vi "AMC e.bloxx Write.vi"(8 "error in (no error)":errorcluster, 9 "Module Command":string, 10 "Module Address":i32, 11 "VISA Resource Name":refnum<visa-resource-name>) -> (0 "error out":errorcluster, 3 "VISA Resource Name out":refnum<visa-resource-name>)   [LabVIEW 2016]
doc: "<B>AMC - Analytik & Messtechnik GmbH Chemnitz</B>\n\nLabVIEW Drivers for e.bloxx series from Gantner Instruments\n\nThis VI is a driver subroutine and should not be used in an application. It assembles a module command string out of the parameters and writes it to the serial interface specified in <B>VISA Resource Name</B>."
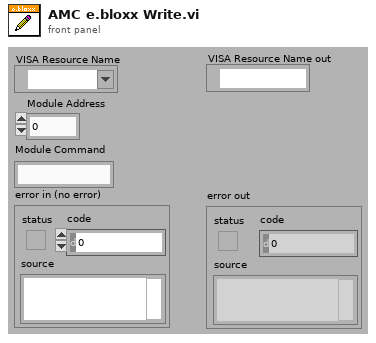
[diagram p1: front panel]
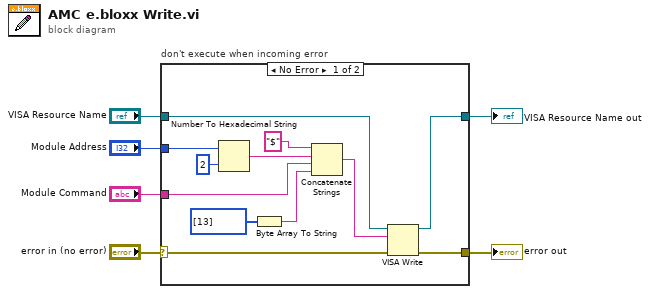
[diagram p0: block diagram]
diagram:
  n1 = case "don't execute when incoming error" shown="No Error" "error in (no error)" {
    selector: "error in (no error)" -> [w18 w20]
    tunnel: [w7 w20] -> w5
    tunnel: "VISA Resource Name" -> [w9 w19]
    tunnel: "Module Command" -> [w12 _]
    tunnel: "Module Address" -> [w17 _]
    tunnel: [w8 w19] -> w1
    frame No Error {
      n2 = Number To Hexadecimal String(1:i16 2 ("width (-)"), 2:w17) -> (0:w13:string)
      n3 = Byte Array To String(unsigned byte array=u8[] [13]) -> (string=w11:string)
      n4 = Concatenate Strings("$", w13, w12, w11) -> (w10:string)
      n5 = VISA Write(VISA resource name=w9, write buffer=w10, error in (no error)=w18) -> (VISA resource name out=w8:refnum<visa-resource-name>, error out=w7:errorcluster)  [unwired: 1 out]
    }
    frame Error {
    }
  }
  "error out" <- w5
  "VISA Resource Name out" <- w1
